vi "CalibrationImageLoadPrompt.vi"() -> (0 "cancel?":bool, 3 "selected path":path)   [LabVIEW 2024]
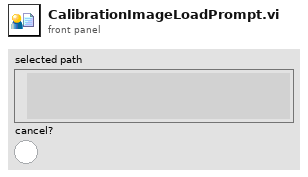
[diagram p1: front panel]
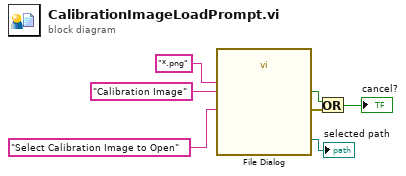
[diagram p0: block diagram]
diagram:
  n1 = call "File Dialog"("prompt"="Select Calibration Image to Open", "pattern (all files)"="*.png", "pattern label"="Calibration Image") -> ("selected path"=→"selected path":path, "cancelled"=w6:bool, "error out"=w7:errorcluster)  [unwired: 9 in, 1 out]
  n2 = Or(x=w6, y=w7) -> (x .or. y?=→"cancel?":bool)
